vi "Column Names.vi"(11 "Optional Save":string[][](array[string])) -> (3 "Output":string)   [LabVIEW 2017]
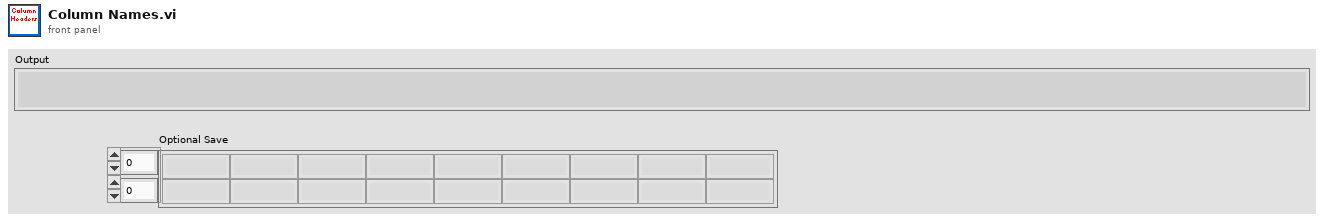
[diagram p1: front panel]
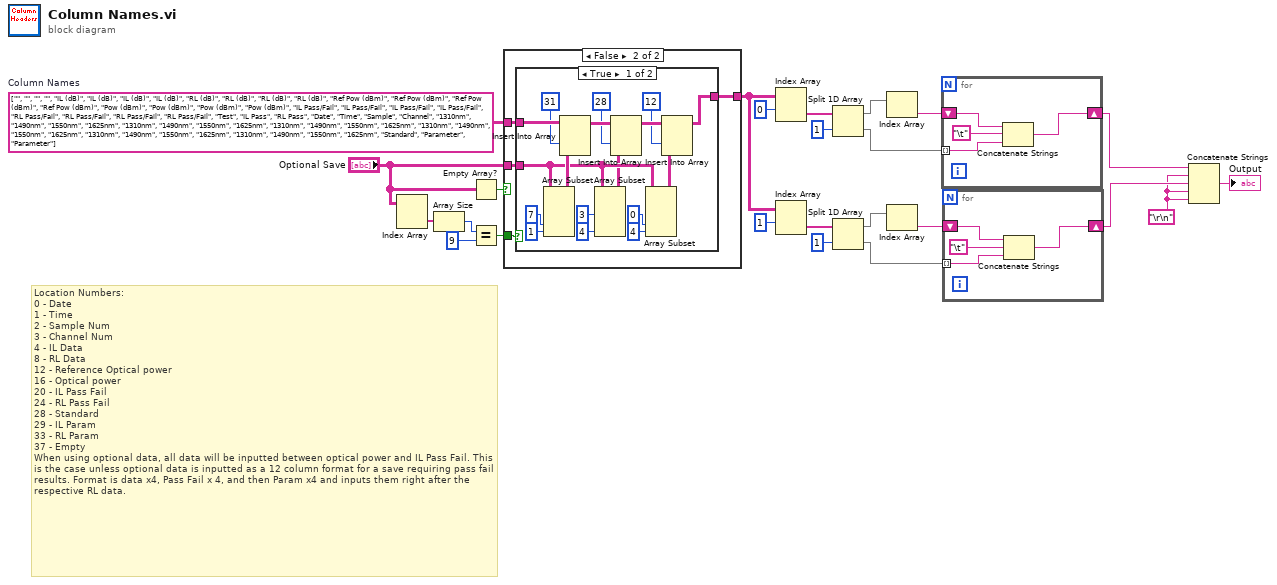
[diagram p0: block diagram]
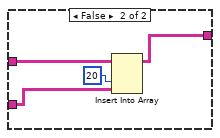
[diagram p3: hidden frame]
diagram:
  w21 = "\r\n"
  w8 = string[][] [["", "", "", "", "IL (dB)", "IL (dB)", "IL (dB)", "IL (dB)", "RL (dB)", "RL (dB)", "RL (dB)", "RL (dB)", "Ref Pow (dBm)", "Ref Pow (dBm)", "Ref Pow (dBm)", "Ref Pow (dBm)", "Pow (dBm)", "Pow (dBm)", "Pow (dBm)", "Pow (dBm)", "IL Pass/Fail", "IL Pass/Fail", "IL Pass/Fail", "IL Pass/Fail", "RL Pass/Fail", "RL Pass/Fail", "RL Pass/Fail", "RL Pass/Fail", "Test", "IL Pass", "RL Pass"], ["Date", "Time", "Sample", "Channel", "1310nm", "1490nm", "1550nm", "1625nm", "1310nm", "1490nm", "1550nm", "1625nm", "1310nm", "1490nm", "1550nm", "1625nm", "1310nm", "1490nm", "1550nm", "1625nm", "1310nm", "1490nm", "1550nm", "1625nm", "1310nm", "1490nm", "1550nm", "1625nm", "Standard", "Parameter", "Parameter"]]  # Column Names
  # "Location Numbers:\n0 - Date\n1 - Time\n2 - Sample Num\n3 - Channel Num\n4 - IL Data\n8 - RL Data\n12 - Reference Optical power\n16 - Optical power\n20 - IL Pass Fail\n24 - RL Pass Fail\n28 - Standard\n29 - IL Param\n33 - RL Param\n37 - Empty \nWhen using optional data, all data will be inputted between optical power and IL Pass Fail. This is the case unless optional data is inputted as a 12 column format for a save requiring pass fail results. Format is data x4, Pass Fail x 4, and then Param x4 and inputs them right after the respective RL data."
  n1 = Index Array(array="Optional Save") -> (element=w4:string[])  [unwired: 2 in]
  n2 = Array Size(array=w4) -> (size(s)=w5:i32)
  n3 = Empty Array?(array="Optional Save") -> (empty?=w7:bool)
  n4 = Equal?(x=w5, y=9) -> (x = y?=w3:bool)
  n5 = case shown="False" w7 {
    tunnel: w8 -> [w25 w29]
    tunnel: w3 -> [_ w28]
    tunnel: "Optional Save" -> [_ w27]
    tunnel: [w25 w26] -> w1
    frame True {
    }
    frame False {
      n6 = case shown="True" w28 {
        tunnel: w29 -> [w45 w50]
        tunnel: w27 -> [w35 w49]
        tunnel: [w44 w48] -> w26
        frame True {
          n7 = Array Subset(array=w35, index (col)=7 ("index (row)"), length (col)=1 ("index (row)")) -> (w46:string[][])  [unwired: 2 in]
          n8 = Insert Into Array(array=w45, index (col)=31 ("index (row)"), new element=w46) -> (w43:string[][])  [unwired: 1 in]
          n9 = Array Subset(array=w35, index (col)=3 ("index (row)"), length (col)=4 ("index (row)")) -> (w34:string[][])  [unwired: 2 in]
          n10 = Insert Into Array(array=w43, index (col)=28 ("index (row)"), new element=w34) -> (w42:string[][])  [unwired: 1 in]
          n11 = Array Subset(array=w35, index (col)=0 ("index (row)"), length (col)=4 ("index (row)")) -> (w33:string[][])  [unwired: 2 in]
          n12 = Insert Into Array(array=w42, index (col)=12 ("index (row)"), new element=w33) -> (w44:string[][])  [unwired: 1 in]
        }
        frame False {
          n13 = Insert Into Array(array=w50, index (col)=20 ("index (row)"), new element=w49) -> (w48:string[][])  [unwired: 1 in]
        }
      }
    }
  }
  n14 = Index Array(array=w1, index (row)=0) -> (element=w18:string[])  [unwired: 1 in]
  n15 = Index Array(array=w1, index (row)=1) -> (element=w15:string[])  [unwired: 1 in]
  n16 = Split 1D Array(array=w18, index=1) -> (first subarray=w12:string[], second subarray=w14:string[])
  n17 = Split 1D Array(array=w15, index=1) -> (first subarray=w9:string[], second subarray=w13:string[])
  n18 = Index Array(array=w12) -> (element=w11:string)  [unwired: 1 in]
  n19 = Index Array(array=w9) -> (element=w10:string)  [unwired: 1 in]
  n20 = for {
    tunnel: w14 -> [w54] mode=indexing
    shift-right: [w53] -> w23
    shift-left: w11 -> [w52]
    n21 = Concatenate Strings(w52, "\t", w54) -> (w53:string)
  }
  n22 = for {
    tunnel: w13 -> [w58] mode=indexing
    shift-right: [w57] -> w24
    shift-left: w10 -> [w56]
    n23 = Concatenate Strings(w56, "\t", w58) -> (w57:string)
  }
  n24 = Concatenate Strings(w23, w21, w24, w21, w21) -> (→"Output":string)
